vi "Get Daemon Connections.vi"(8 "error in (no error)":errorcluster, 11 "Modbus slave in":refnum<class "Modbus Slave.lvclass">) -> (0 "error out":errorcluster, 2 "connections":T1(array[cluster]), 3 "Modbus slave out":refnum<class "Modbus Slave.lvclass">)   [LabVIEW 2021, in "Modbus Slave.lvclass"]
doc: "<B>TCP Connection List</B> returns the information about the TCP connections established to the Modbus slave. This information shows you the IP address and connection error of a Modbus master and whether this Modbus master is connected to the Modbus slave. To get this property, ensure that you wire a TCP Modbus slave to the <B>reference</B> input. Otherwise, LabVIEW returns error code -389106."
uses:
  Modbus Slave.lvclass
  Modbus Slave.lvclass/Modbus Slave.ctl
  Network Protocol/Network Slave/TCP/TCP Slave.lvclass
  Network Protocol/Network Slave/TCP/TCP Slave.lvclass/TCP Slave.ctl
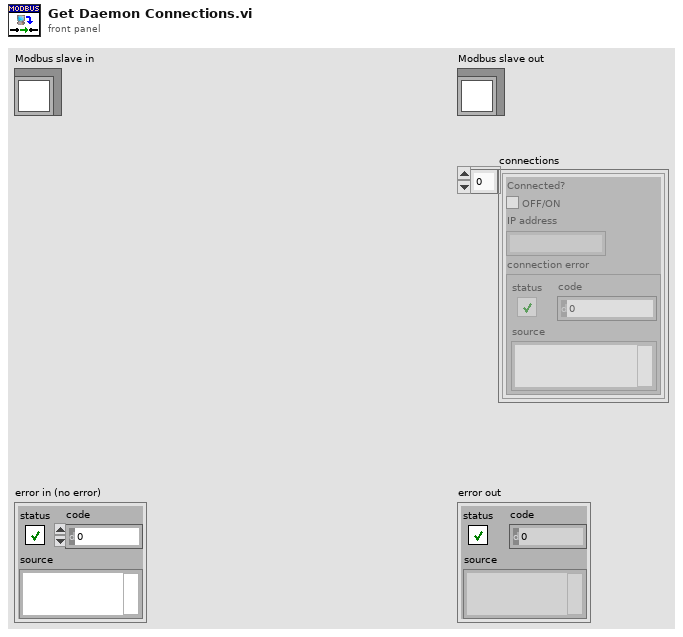
[diagram p1: front panel]
types:
  T1 = cluster{"Connected?":bool, "IP address":string, "connection error":errorcluster}[]
  T2 = typedef "TCP Slave.lvclass/Connection.ctl" = cluster{"Connected?":bool, "IP address":string, "connection error":errorcluster}
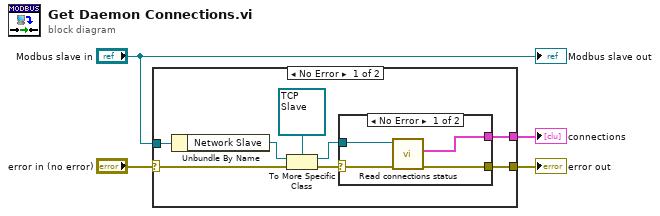
[diagram p0: block diagram]
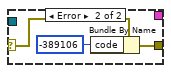
[diagram p2: hidden frame]
diagram:
  n1 = case shown="No Error" "error in (no error)" {
    selector: "error in (no error)" -> [w5 w20]
    tunnel: [w10 _] -> w2
    tunnel: [w9 w20] -> w3
    tunnel: "Modbus slave in" -> [w7 _]
    frame No Error {
      n2 = Unbundle By Name(w7) -> ("Network Slave"=w6:refnum<class "Network Slave.lvclass">)
      n3 = To More Specific Class(target class=refnum<class "TCP Slave.lvclass"> refnum ("TCP Slave"), reference=w6, error in=w5) -> (specific class reference=w11:refnum<class "TCP Slave.lvclass">, error out=w12:errorcluster)
      n4 = case shown="No Error" w12 {
        selector: w12 -> [w15 w19]
        tunnel: w11 -> [w16 _]
        tunnel: [w13 _] -> w10
        tunnel: [w14 w18] -> w9
        frame No Error {
          n5 = call "Read connections status.vi"("error in (no error)"=w15, "TCP Slave in"=w16) -> ("error out"=w14:errorcluster, "Connections"=w13:T2[])  [unwired: 7 in, 1 out]
        }
        frame Error {
          n6 = Bundle By Name(cluster=w19, "code"=-389106) -> (w18:errorcluster)
        }
      }
    }
    frame Error {
    }
  }
  "error out" <- w3
  "connections" <- w2
  "Modbus slave out" <- "Modbus slave in"
